vi "Open.vi"(11 "Serial Number":string="30430219") -> (2 "Handle Number":i32, 3 "SN OUT":string)   [LabVIEW 2022 SP3]
doc: "HANDLE H11890API __stdcall H11890Open(char* cSerialNumber);"
uses:
  EXE/data/H11890api.dll
panel:
  in  "OK":bool
  # "Input serial number <H11890 series>"
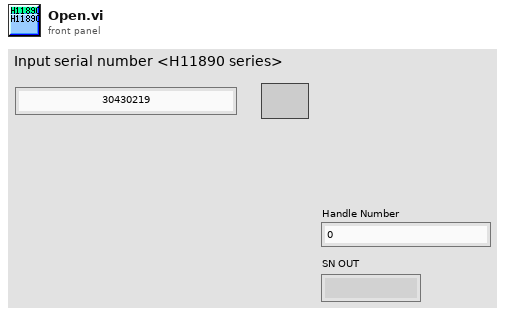
[diagram p1: front panel]
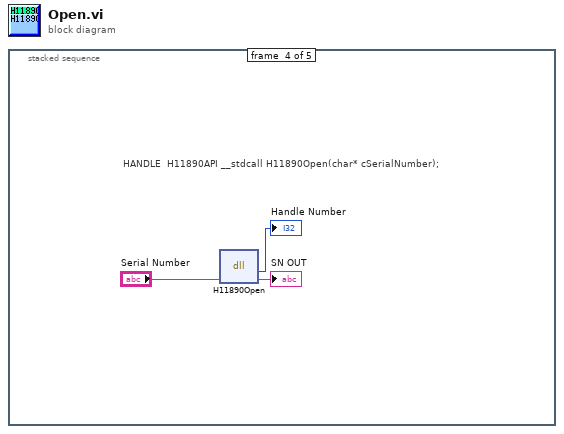
[diagram p0: block diagram]
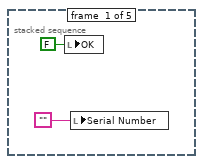
[diagram p2: hidden frame]
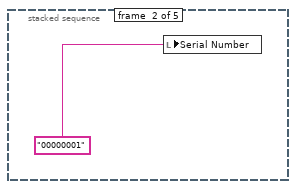
[diagram p3: hidden frame]
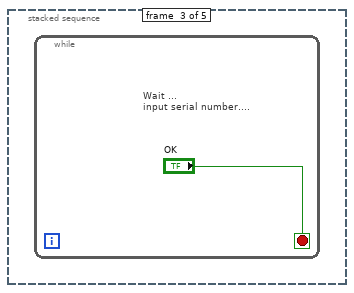
[diagram p4: hidden frame]
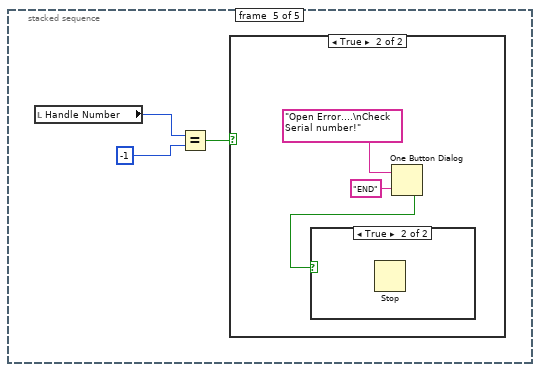
[diagram p5: hidden frame]
diagram:
  n1 = stacked-sequence {
    frame #0 {
      n2 = local write "OK"(FALSE ("OK")) -> ()
      n3 = local write "Serial Number"("") -> ()
    }
    frame #1 {
      n4 = local write "Serial Number"("00000001" ("Serial Number")) -> ()
    }
    frame #2 {
      n5 = while {
        stop <- "OK" stop-if-true
        # "Wait ...\ninput serial number...."
      }
    }
    frame #3 {
      # "HANDLE\t\tH11890API __stdcall H11890Open(char* cSerialNumber);"
      n6 = dll-call lib="C:/Users/Public/OneDrive/Desktop/PMT program/SampleCodeLabView/EXE/data/H11890api.dll" fn="H11890Open"("cSerialNumber"="Serial Number") -> ("Hnadle"=→"Handle Number":i32, "cSerialNumber"=→"SN OUT":string)  [unwired: 3 in, 2 out]
    }
    frame #4 {
      n7 = local read "Handle Number"() -> (w10:i32)
      n8 = Equal?(x=w10, y=-1) -> (x = y?=w8:bool)
      n9 = case shown="True" w8 {
        frame False {
        }
        frame True {
          n10 = One Button Dialog(message="Open Error....\nCheck Serial number!" ("メッセージ"), button name ("OK")="END" ("ボタン名（\"OK\"）")) -> (true=w11:bool)
          n11 = case shown="True" w11 {
            frame False {
            }
            frame True {
              n12 = Stop() -> ()  [unwired: 1 in]
            }
          }
        }
      }
    }
  }
